vi "Init Loop.vi"(4 "Not found":refnum<class "CConfig Query.lvclass">, 6 "Found":refnum<class "CConfig Query.lvclass">, 8 "error in (no error)":errorcluster, 11 "Loop Query":refnum<class "Loop Query.lvclass">) -> (0 "error out":errorcluster, 3 "Loop Query":refnum<class "Loop Query.lvclass">)   [LabVIEW 2013, in "Loop Query.lvclass"]
doc: "Copyright 2018, Carya Automatisering, Wiebe Walstra."
uses:
  Loop Query.lvclass
  CConfig Query.lvclass
  Loop Query.lvclass/Loop Query.ctl
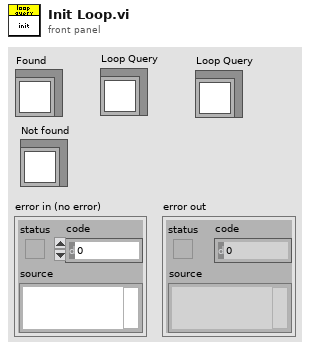
[diagram p1: front panel]
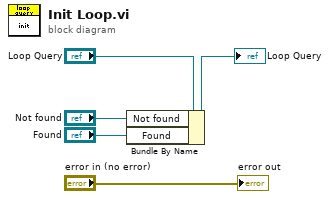
[diagram p0: block diagram]
diagram:
  n1 = Bundle By Name(cluster="Loop Query", "Not found"="Not found", "Found"="Found") -> (→"Loop Query":refnum<class "Loop Query.lvclass">)
  "error out" <- "error in (no error)"
